vi "Microscope.GetDependenciesPublicEvents.vi"(8 "error in (no error)":errorcluster, 11 "Microscope":refnum<class "Microscope.lvclass">) -> (0 "error out":errorcluster, 1 "XYStage Public Events":T2, 2 "Camera Public Events":T1, 3 "Microscope out":refnum<class "Microscope.lvclass">)   [LabVIEW 2015, in "Microscope.lvclass"]
doc: "---------------------------------------------------------------\nJKI State Machine Objects™\nhttp://jki.net/state-machine-objects/\nCopyright (C) 2005-2015, JKI <info@jki.net>\nALL RIGHTS RESERVEDJKI State Machine Objects (SMO) 1.0.0.5\nJKI - JKI\nCopyright (c) 2016, JKI"
uses:
  Microscope.lvclass
  XYStage/Typedefs/PublicEvents--Cluster.ctl
  XYStage/Typedefs/(real)Coords--Cluster.ctl
  XYStage/Typedefs/PublicEvents--XYStage.UpdatedNamedPosition.ctl
  Camera/Typedefs/PublicEvents--Cluster.ctl
  Camera/Camera.lvclass
  XYStage/XYStage.lvclass
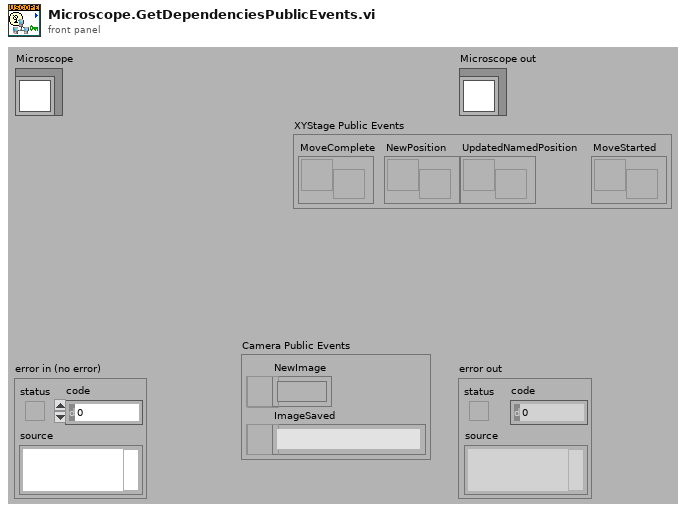
[diagram p1: front panel]
types:
  T1 = typedef "Camera.lvclass/PublicEvents--Cluster.ctl" = cluster{"NewImage":refnum<user-event>, "ImageSaved":refnum<user-event>}
  T2 = typedef "XYStage.lvclass/PublicEvents--Cluster.ctl" = cluster{"MoveComplete":refnum<user-event>, "NewPosition":refnum<user-event>, "UpdatedNamedPosition":refnum<user-event>, "MoveStarted":refnum<user-event>}
  T3 = typedef "Microscope.lvclass/Dependencies--Cluster.ctl" = cluster{"XYStage":refnum<class "XYStage.lvclass">, "Camera":refnum<class "Camera.lvclass">}
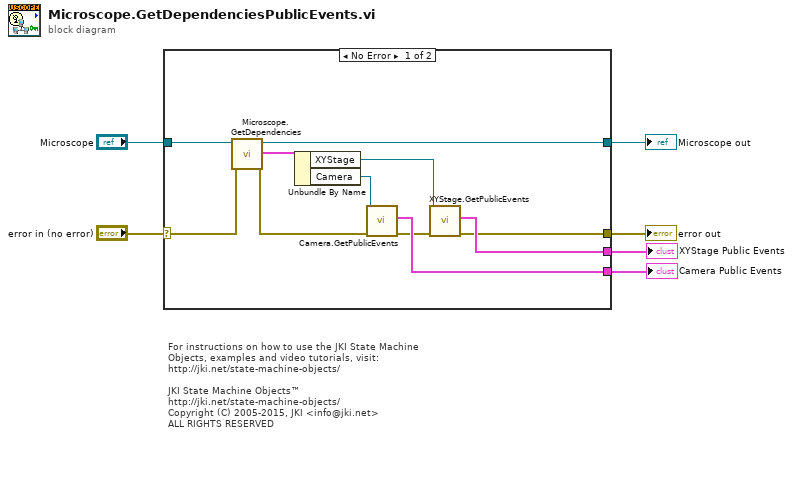
[diagram p0: block diagram]
diagram:
  # "For instructions on how to use the JKI State Machine Objects, examples and video tutorials, visit:\nhttp://jki.net/state-machine-objects/\n\nJKI State Machine Objects™\nhttp://jki.net/state-machine-objects/\nCopyright (C) 2005-2015, JKI <info@jki.net>\nALL RIGHTS RESERVED"
  n1 = case shown="No Error" "error in (no error)" {
    selector: "error in (no error)" -> [w16 w18]
    tunnel: "Microscope" -> [w17 w19]
    tunnel: [w8 w18] -> w5
    tunnel: [w15 w19] -> w4
    tunnel: [w12 _] -> w2
    tunnel: [w11 _] -> w1
    frame No Error {
      n2 = call "Microscope.GetDependencies.vi"("error in (no error)"=w16, "Microscope"=w17) -> ("error out"=w9:errorcluster, "Dependencies"=w14:T3, "Microscope out"=w15:refnum<class "Microscope.lvclass">)  [unwired: 7 in]
      n3 = Unbundle By Name(w14) -> ("XYStage"=w7:refnum<class "XYStage.lvclass">, "Camera"=w13:refnum<class "Camera.lvclass">)
      n4 = call "Camera.GetPublicEvents.vi"("error in (no error)"=w9, "Camera"=w13) -> ("error out"=w10:errorcluster, "Camera Public Events"=w11:T1)  [unwired: 7 in, 1 out]
      n5 = call "XYStage.GetPublicEvents.vi"("error in (no error)"=w10, "XYStage"=w7) -> ("error out"=w8:errorcluster, "XYStage Public Events"=w12:T2)  [unwired: 7 in, 1 out]
    }
    frame Error {
    }
  }
  "error out" <- w5
  "Microscope out" <- w4
  "XYStage Public Events" <- w2
  "Camera Public Events" <- w1
